vi "UI_sendSimpleMessage.vi"(5 "Notif T/O":i32=250, 6 "notifier":refnum<notifier>, 7 "Wait for Response":bool, 8 "error in (no error)":errorcluster, 10 "Command":string, 11 "Queue Bus":T1) -> (0 "error out":errorcluster, 2 "payload":variant, 3 "Queue Bus OUT":T1)   [LabVIEW 2020]
uses:
  Typedefs/queueBus.ctl
  Typedefs/communicationData.ctl
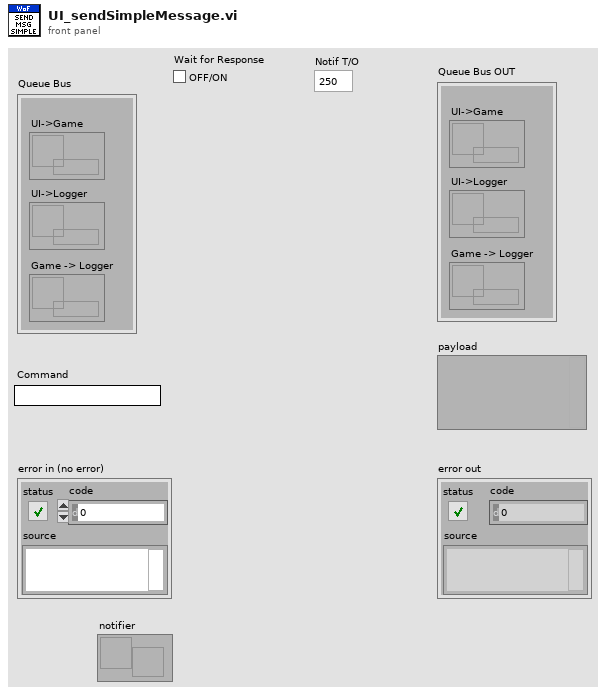
[diagram p1: front panel]
types:
  T1 = typedef "queueBus.ctl" = cluster{"UI->Game":refnum<queue>, "UI->Logger":refnum<queue>, "Game -> Logger":refnum<queue>}
  T2 = typedef "communicationData.ctl" = cluster{"command":string, "payload":variant, "response":variant}
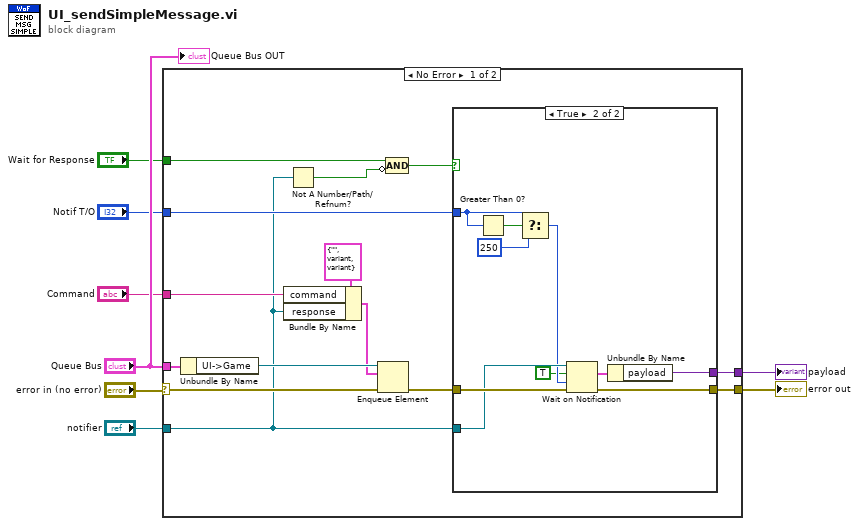
[diagram p0: block diagram]
diagram:
  n1 = case shown="No Error" "error in (no error)" {
    selector: "error in (no error)" -> [w20 w34]
    tunnel: [w14 w34] -> w8
    tunnel: "notifier" -> [w9 _]
    tunnel: "Queue Bus" -> [w22 _]
    tunnel: "Command" -> [w18 _]
    tunnel: "Wait for Response" -> [w16 _]
    tunnel: "Notif T/O" -> [w13 _]
    tunnel: [w12 _] -> w1
    frame No Error {
      n2 = Unbundle By Name(w22) -> ("UI->Game"=w21:refnum<queue>)
      n3 = Bundle By Name(cluster=T2 {"command"="", "payload"=variant, "response"=variant} ("communication"), "command"=w18, "response"=w9) -> (w17:T2)
      n4 = Not A Number/Path/Refnum?(number/path/refnum=w9) -> (NaN/Path/Refnum?=w10:bool)
      n5 = Enqueue Element(queue=w21, element=w17, error in (no error)=w20) -> (error out=w15:errorcluster)  [unwired: 1 in, 2 out]
      n6 = Compound Arithmetic op=AND(w16, invert w10) -> (w11:bool)
      n7 = case shown="True" w11 {
        tunnel: w15 -> [w23 w33]
        tunnel: [w23 w32] -> w14
        tunnel: w9 -> [_ w31]
        tunnel: w13 -> [_ w29]
        tunnel: [_ w24] -> w12
        frame False {
        }
        frame True {
          n8 = Greater Than 0?(x=w29) -> (x > 0?=w30:bool)
          n9 = Select(t=w29, s=w30, f=250) -> (s? t:f=w27:i32)
          n10 = Wait on Notification(notifier=w31, ignore previous (F)=TRUE, timeout in ms (-1)=w27, error in (no error)=w33) -> (notification=w25:T2, error out=w32:errorcluster)  [unwired: 2 out]
          n11 = Unbundle By Name(w25) -> ("payload"=w24:variant)
        }
      }
    }
    frame Error {
    }
  }
  "error out" <- w8
  "payload" <- w1
  "Queue Bus OUT" <- "Queue Bus"
